vi "value_to_index.vi"(2 "values":dbl[](array[numeric])=[2.0, 2.0, 4.0, 3.0], 3 "lookup array":dbl[](array[numeric])=[3.0, 2.0, 4.0]) -> (1 "indices":i64[](array[numeric])=[1, 1, 2, 0])   [LabVIEW 2014]
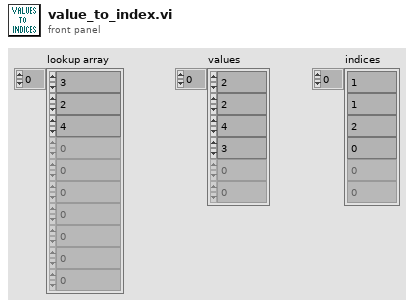
[diagram p1: front panel]
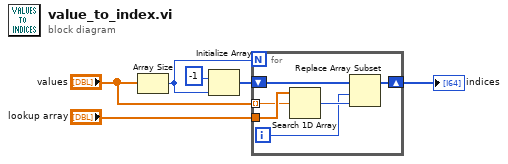
[diagram p0: block diagram]
diagram:
  n1 = Array Size(array="values") -> (size(s)=w1:i32)
  n2 = Initialize Array(i64 -1 ("element"), w1) -> (w4:i64[])
  n3 = for {
    N: w1 -> [_]
    tunnel: "lookup array" -> [w12]
    shift-right: [w9] -> w6
    shift-left: w4 -> [w11]
    tunnel: "values" -> [w10] mode=indexing
    i -> [w7]
    n4 = Search 1D Array(1D array=w12, element=w10) -> (index of element=w8:i32)  [unwired: 1 in]
    n5 = Replace Array Subset(array=w11, new element=w8, index=w7) -> (w9:i64[])
  }
  "indices" <- w6
